vi "Serial Read.vi"(8 "error in (no error)":errorcluster, 10 "Connection ID":i32, 11 "Gantry in":refnum<class "Gantry.lvclass">) -> (0 "error out":errorcluster, 2 "read buffer":string, 3 "Gantry out":refnum<class "Gantry.lvclass">)   [LabVIEW 2023, in "Gantry.lvclass"]
uses:
  Gantry.lvclass
  Gantry.lvclass/Gantry.ctl
  <vilib>/Utility/error.llb/whitespace.ctl
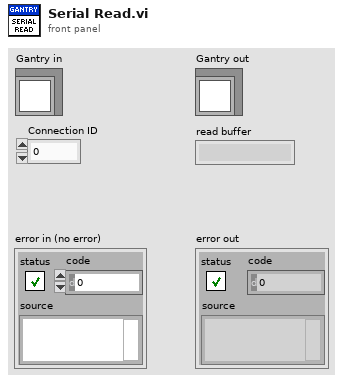
[diagram p1: front panel]
types:
  T1 = typedef "whitespace.ctl" = u16
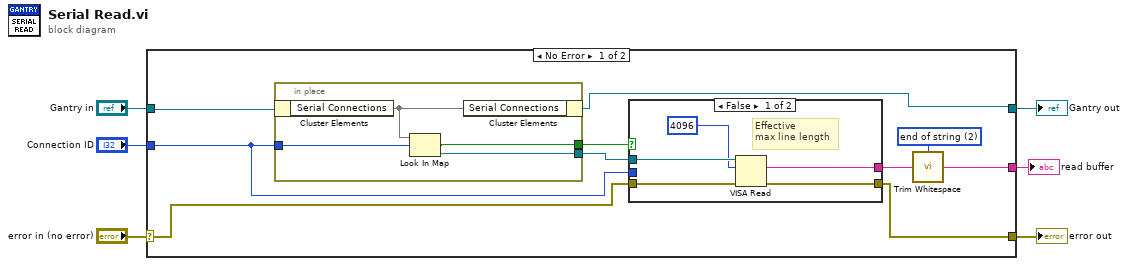
[diagram p0: block diagram]
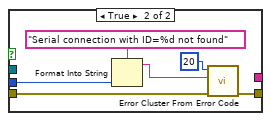
[diagram p2: hidden frame]
diagram:
  n1 = case shown="No Error" "error in (no error)" {
    selector: "error in (no error)" -> [w13 w33]
    tunnel: [w10 w33] -> w5
    tunnel: [w11 w32] -> w3
    tunnel: "Gantry in" -> [w14 w32]
    tunnel: "Connection ID" -> [w12 _]
    tunnel: [w8 _] -> w1
    frame No Error {
      w7 = T1 2 items=["both", "start of string", "end of string"] ("location (both)")
      n2 = in-place {
        in-place-border: w12 -> [w31]
        in-place-border: [w30] -> w15
        in-place-border: [w29] -> w16
        n3 = in-place-cluster #1(w14) -> ("Serial Connections"=w28:map{i32, refnum<visa-resource-name>})
        n4 = Look In Map(map=w28, key=w31) -> (key not found?=w29:bool, value=w30:refnum<visa-resource-name>)  [unwired: 1 in]
        n5 = in-place-cluster #1("Serial Connections"=w28) -> (w11:refnum<class "Gantry.lvclass">)
      }
      n6 = case shown="False" w16 {
        tunnel: w15 -> [w21 _]
        tunnel: w13 -> [w20 w27]
        tunnel: w12 -> [_ w24]
        tunnel: [w19 w22] -> w10
        tunnel: [w17 _] -> w9
        frame False {
          # "Effective\nmax line length"
          n7 = VISA Read(VISA resource name=w21, byte count=u32 4096, error in (no error)=w20) -> (read buffer=w17:string, error out=w19:errorcluster)  [unwired: 2 out]
        }
        frame True {
          n8 = Format Into String(format string="Serial connection with ID=%d not found", w24) -> (resulting string=w23:string)  [unwired: 2 in, 1 out]
          n9 = call <vilib>:"Error Cluster From Error Code.vi"("error in (no error)"=w27, "error message (\"\")"=w23, "error code (0)"=20) -> ("error out"=w22:errorcluster)  [unwired: 6 in]
        }
      }
      n10 = call <vilib>:"Trim Whitespace.vi"("string"=w9, "location (both)"=w7) -> ("trimmed string"=w8:string)
    }
    frame Error {
    }
  }
  "error out" <- w5
  "Gantry out" <- w3
  "read buffer" <- w1
